vi "SS_Channel_and_Sample_Number.vi"(6 "Main Cluster IN":T1, 7 "FPGA Info IN":T3, 8 "Error In":errorcluster, 9 "RT Duration":string, 10 "DATA":dbl[][](array[numeric]), 11 "Info In":string="\nWaiting for TimerScope Trigger\n- IN: SS TimerScope Trigger\n- OUT: SET SS ThermoRec Received Trigger\nPulse Number is 231123\nPulse Type is 4\n\nDuration (s) is  2.000000\nDelay (s)  is  1.000000\nScan Period (ms) is  15\nNumber of Samples is  134\n\nDelay Started\nDelay Complete\nExternal Measurement of Delay (s): 1.000000\nACQUIRING DATA") -> (0 "Error Out":errorcluster, 3 "Info Out":string="\nWaiting for TimerScope Trigger\n- IN: SS TimerScope Trigger\n- OUT: SET SS ThermoRec Received Trigger\nPulse Number is 231123\nPulse Type is 4\n\nDuration (s) is  2.000000\nDelay (s)  is  1.000000\nScan Period (ms) is  15\nNumber of Samples is  134\n\nDelay Started\nDelay Complete\nExternal Measurement of Delay (s): 1.000000\nACQUIRING DATA", 4 "Main Cluster OUT":T1)   [LabVIEW 2016]
uses:
  Control/Control_Main.ctl
  Control/Control_ModuleArray.ctl
panel:
  in  "Tab Control":enum32{"IN", "OUT", "SubVI Info"}(tab)
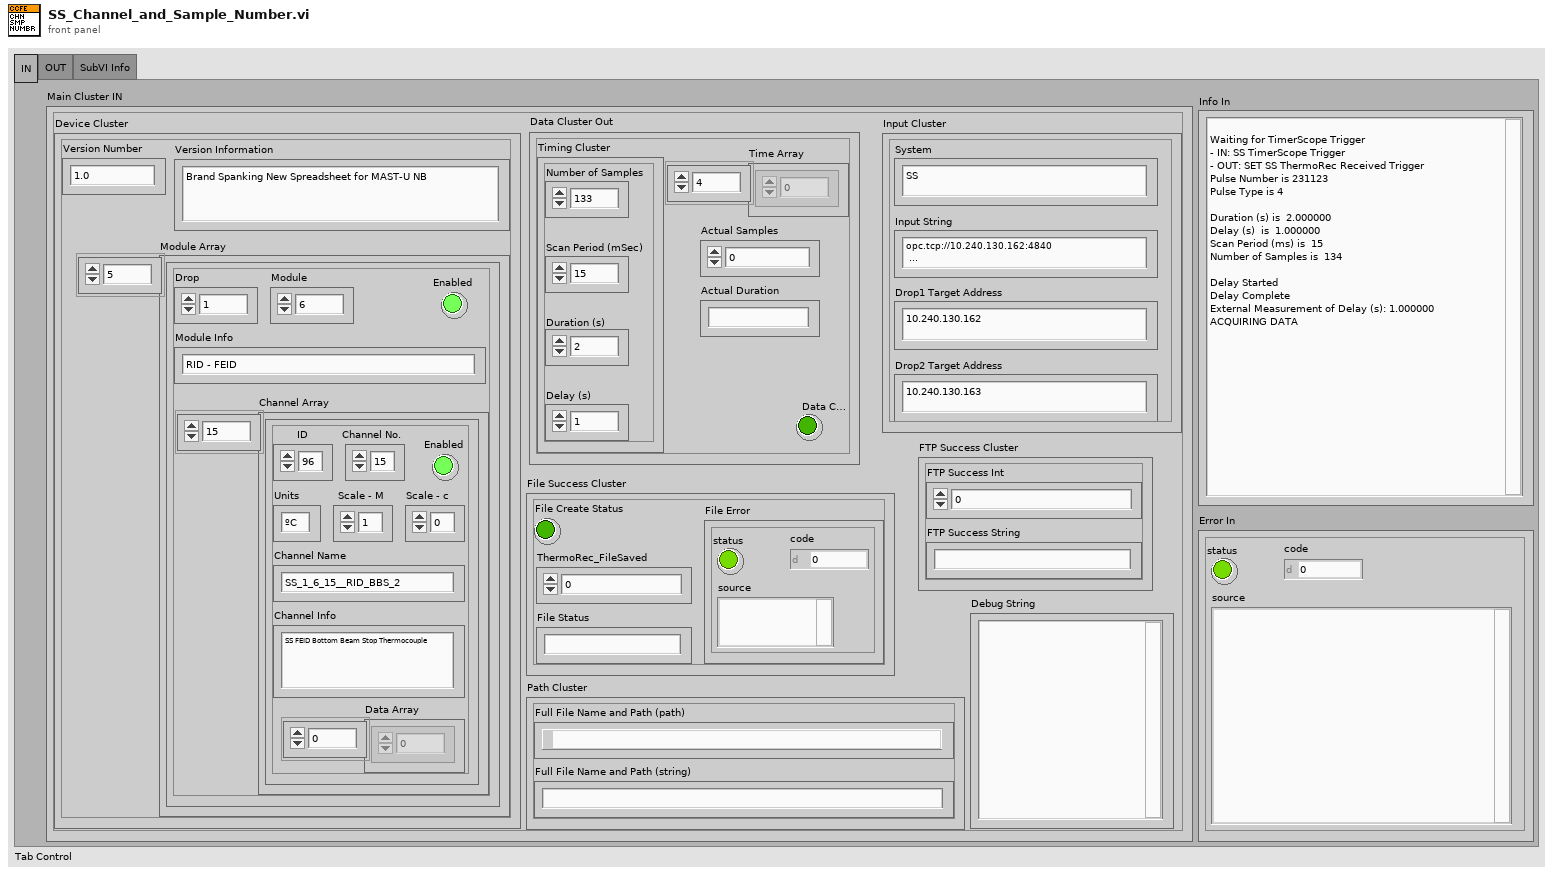
[diagram p1: front panel]
types:
  T1 = typedef "Control_Main.ctl" = cluster{"Device Cluster":cluster{"Module Array":T2, "Version Number":string, "Version Information":string}, "Input Cluster":cluster{"Input String":string, "Drop1 Target Address":string, "Drop2 Target Address":string, "System":string}, "Data Cluster Out":cluster{"Timing Cluster":cluster{"Number of Samples":i32, "Scan Period (mSec)":u32, "Duration (s)":dbl, "Delay (s)":dbl}, "Time Array":dbl[], "Actual Samples":i32, "Actual Duration":string, "Data Collection Error":bool}, "Path Cluster":cluster{"Full File Name and Path (path)":path, "Full File Name and Path (string)":string}, "File Success Cluster":cluster{"ThermoRec_FileSaved":i32, "File Create Status":bool, "File Error":errorcluster, "File Status":string}, "FTP Success Cluster":cluster{"FTP Success Int":i32, "FTP Success String":string}, "Debug String":string}
  T2 = typedef "Control_ModuleArray.ctl" = cluster{"Drop":i32, "Module":i32, "Module Info":string, "Enabled":bool, "Channel Array":cluster{"ID":i32, "Channel No.":i32, "Enabled":bool, "Channel Name":string, "Channel Info":string, "Units":string, "Scale - M":dbl, "Scale - c":dbl, "Data Array":dbl[]}[]}[]
  T3 = cluster{"Drop0":cluster{"Actual Duration (ms)":i32, "Actual Number of Samples":i32}, "Drop1":cluster{"Actual Duration (ms)":i32, "Actual Number of Samples":i32}}
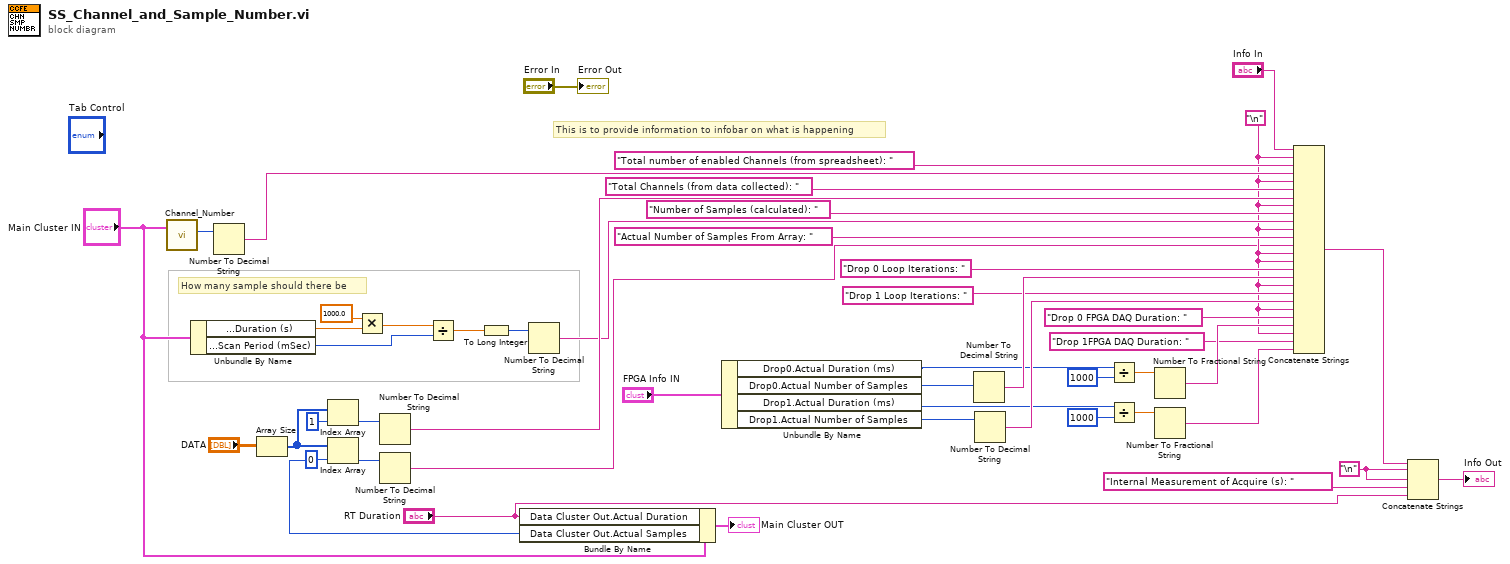
[diagram p0: block diagram]
diagram:
  w7 = "\n"
  w4 = "\n"
  # "This is to provide information to infobar on what is happening"
  # "How many sample should there be"
  n1 = call "Channel_Number.vi"("Main Cluster IN"="Main Cluster IN") -> ("Total Number of Channels"=w16:i32)  [unwired: 8 in, 2 out]
  n2 = Unbundle By Name("Main Cluster IN") -> ("Data Cluster Out.Timing Cluster.Duration (s)"=w48:dbl, "Data Cluster Out.Timing Cluster.Scan Period (mSec)"=w45:u32)
  n3 = Number To Decimal String(number=w16) -> (decimal integer string=w15:string)  [unwired: 1 in]
  n4 = Array Size(array="DATA") -> (size(s)=w39:i32[])
  n5 = Index Array(array=w39, index=1) -> (element=w42:i32)
  n6 = Index Array(array=w39, index=0) -> (element=w21:i32)
  n7 = Multiply(x=1000.0, y=w48) -> (x*y=w46:dbl)
  n8 = Number To Decimal String(number=w42) -> (decimal integer string=w36:string)  [unwired: 1 in]
  n9 = Number To Decimal String(number=w21) -> (decimal integer string=w1:string)  [unwired: 1 in]
  n10 = Divide(x=w46, y=w45) -> (x/y=w44:dbl)
  n11 = To Long Integer(number=w44) -> (32bit integer=w43:i32)
  n12 = Bundle By Name(cluster="Main Cluster IN", "Data Cluster Out.Actual Duration"="RT Duration", "Data Cluster Out.Actual Samples"=w21) -> (→"Main Cluster OUT":T1)
  n13 = Number To Decimal String(number=w43) -> (decimal integer string=w34:string)  [unwired: 1 in]
  n14 = Unbundle By Name("FPGA Info IN") -> ("Drop0.Actual Duration (ms)"=w13:i32, "Drop0.Actual Number of Samples"=w12:i32, "Drop1.Actual Duration (ms)"=w11:i32, "Drop1.Actual Number of Samples"=w10:i32)
  n15 = Number To Decimal String(number=w12) -> (decimal integer string=w28:string)  [unwired: 1 in]
  n16 = Number To Decimal String(number=w10) -> (decimal integer string=w26:string)  [unwired: 1 in]
  n17 = Divide(x=w13, y=u32 1000) -> (x/y=w24:dbl)
  n18 = Divide(x=w11, y=u32 1000) -> (x/y=w22:dbl)
  n19 = Number To Fractional String(number=w24) -> (F-format string=w5:string)  [unwired: 3 in]
  n20 = Number To Fractional String(number=w22) -> (F-format string=w2:string)  [unwired: 3 in]
  n21 = Concatenate Strings("Info In", w4, "Total number of enabled Channels (from spreadsheet): ", w15, w4, "Total Channels (from data collected): ", w36, w4, "Number of Samples (calculated): ", w34, w4, "Actual Number of Samples From Array: ", w1, w4, w4, "Drop 0 Loop Iterations: ", w28, w4, "Drop 1 Loop Iterations: ", w26, w4, "Drop 0 FPGA DAQ Duration: ", w5, w4, "Drop 1FPGA DAQ Duration: ", w2) -> (w18:string)
  n22 = Concatenate Strings(w18, w7, w7, "Internal Measurement of Acquire (s): ", "RT Duration") -> (→"Info Out":string)
  "Error Out" <- "Error In"
